vi "Initialize.vi"(8 "error in (no error)":errorcluster, 11 "[C] User Management in":refnum<class "[C] User Management.lvclass">) -> (0 "error out":errorcluster, 3 "[C] User Management out":refnum<class "[C] User Management.lvclass">)   [LabVIEW 2020, in "[C] User Management.lvlib" / "[C] User Management.lvclass"]
uses:
  [C] User Management.lvclass
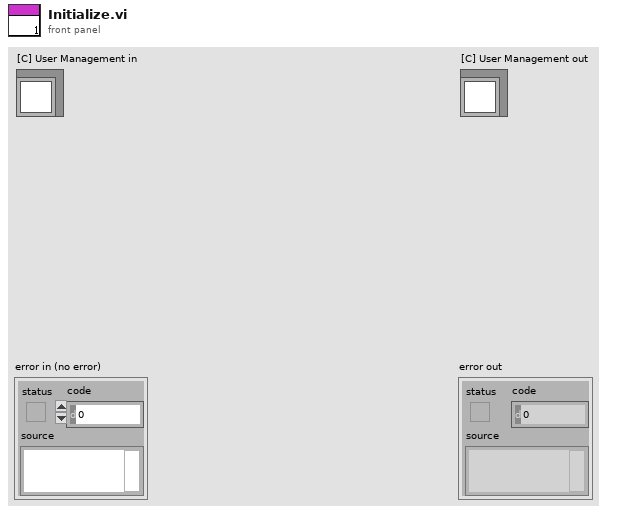
[diagram p1: front panel]
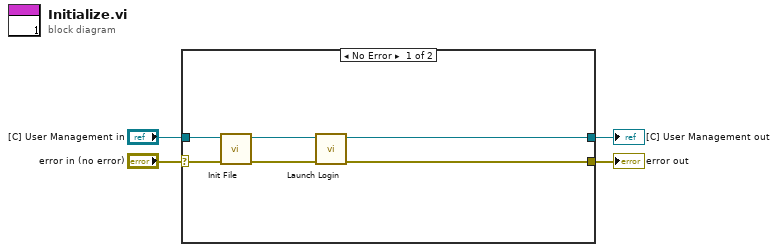
[diagram p0: block diagram]
diagram:
  n1 = case shown="No Error" "error in (no error)" {
    selector: "error in (no error)" -> [w8 w12]
    tunnel: [w9 w12] -> w3
    tunnel: [w10 w11] -> w1
    tunnel: "[C] User Management in" -> [w7 w11]
    frame No Error {
      n2 = call "Init File.vi"("error in (no error)"=w8, "[C] User Management in"=w7) -> ("error out"=w6:errorcluster, "[C] User Management out"=w5:refnum<class "[C] User Management.lvclass">)  [unwired: 8 in]
      n3 = call "Launch Login.vi"("error in (no error)"=w6, "[C] User Management in"=w5) -> ("error out"=w9:errorcluster, "[C] User Management out"=w10:refnum<class "[C] User Management.lvclass">)  [unwired: 8 in]
    }
    frame Error {
    }
  }
  "error out" <- w3
  "[C] User Management out" <- w1
